vi "vision1.vi"(8 "error in":errorcluster) -> (0 "error out":errorcluster)   [LabVIEW 2017]
uses:
  <vilib>/userdefined/High Color/IMAQdx.ctl
  addres.vi
  <vilib>/vision/driver/NI_Vision_Acquisition_Software.lvlib
panel:
  out "color":string
  out "number":string
  out "Image":T1(plugin-control)
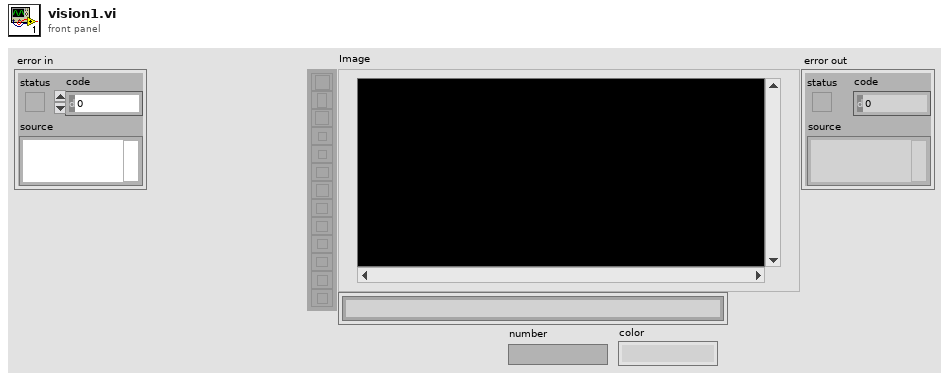
[diagram p1: front panel]
types:
  T1 = typedef "IMAQ Image.ctl" = refnum<image>
  T2 = typedef "IMAQdx.ctl" = refnum<k21>
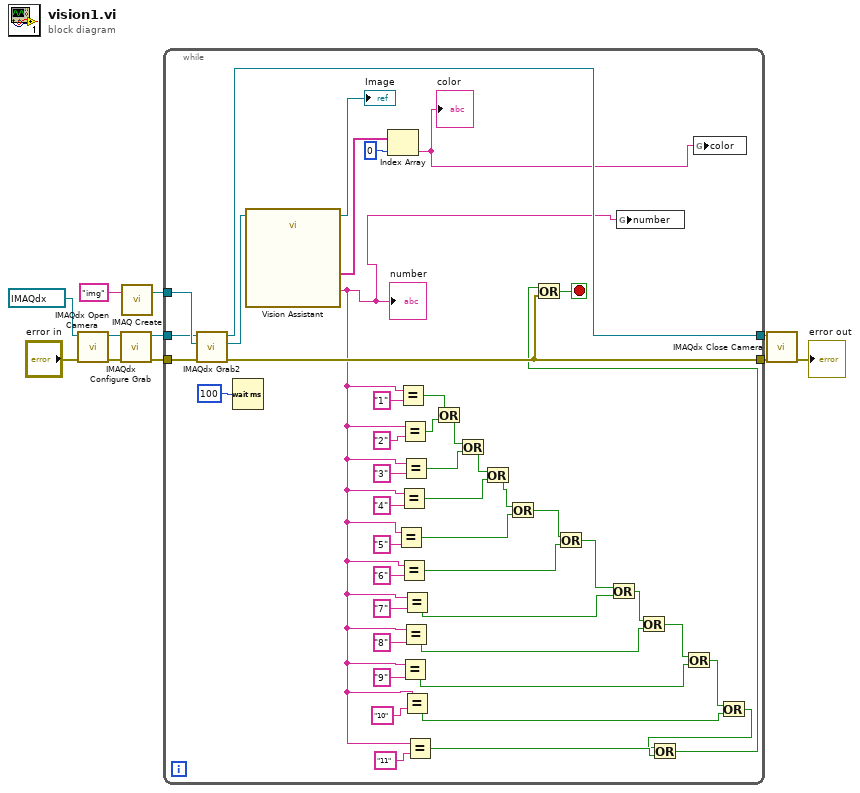
[diagram p0: block diagram]
diagram:
  n1 = call <vilib>:"IMAQdx Open Camera.vi"("error in"="error in", "Session In"=T2 "cam0") -> ("error out"=w8:errorcluster, "Session Out"=w5:T2)  [unwired: 8 in]
  n2 = call <vilib>:"IMAQdx Configure Grab.vi"("error in"=w8, "Session In"=w5) -> ("error out"=w7:errorcluster, "Session Out"=w4:T2)  [unwired: 8 in]
  n3 = call "IMAQ Create"("Image Name"="img") -> ("New Image"=w6:T1)  [unwired: 4 in, 1 out]
  n4 = while {
    tunnel: w7 -> [w56]
    tunnel: w6 -> [w55]
    tunnel: w4 -> [w54]
    tunnel: [w53] -> w3
    tunnel: [w47] -> w11
    stop <- w46 stop-if-true
    n5 = call <vilib>:"IMAQdx Grab2.vi"("error in"=w56, "Image In"=w55, "Session In"=w54) -> ("error out"=w47:errorcluster, "Image Out"=w52:T1, "Session Out"=w53:T2)  [unwired: 5 in, 1 out]
    n6 = Wait (ms)(milliseconds to wait=u32 100) -> ()  [unwired: 1 out]
    n7 = call "Vision Assistant"("Image In"=w52) -> ("Image Out"=→"Image":T1, "String (OCR/OCV 1)"=w15:string, "Classes (Color Classification 1)"=w49:string[])  [unwired: 23 in, 1 out]
    "number" <- w15
    n8 = Index Array(array=w49, index=0) -> (element=w17:string)
    "color" <- w17
    n9 = Equal?(x=w15, y="5") -> (x = y?=w35:bool)
    n10 = Equal?(x=w15, y="1") -> (x = y?=w28:bool)
    n11 = Equal?(x=w15, y="4") -> (x = y?=w33:bool)
    n12 = Equal?(x=w15, y="6") -> (x = y?=w37:bool)
    n13 = Equal?(x=w15, y="2") -> (x = y?=w29:bool)
    n14 = Equal?(x=w15, y="9") -> (x = y?=w43:bool)
    n15 = Equal?(x=w15, y="3") -> (x = y?=w31:bool)
    n16 = Equal?(x=w15, y="8") -> (x = y?=w40:bool)
    n17 = Equal?(x=w15, y="7") -> (x = y?=w39:bool)
    n18 = Equal?(x=w15, y="10") -> (x = y?=w45:bool)
    n19 = Equal?(x=w15, y="11") -> (x = y?=w14:bool)
    n20 = Or(x=w28, y=w29) -> (x .or. y?=w30:bool)
    n21 = Or(x=w30, y=w31) -> (x .or. y?=w32:bool)
    n22 = Or(x=w32, y=w33) -> (x .or. y?=w34:bool)
    n23 = Or(x=w34, y=w35) -> (x .or. y?=w36:bool)
    n24 = Or(x=w36, y=w37) -> (x .or. y?=w38:bool)
    n25 = Or(x=w38, y=w39) -> (x .or. y?=w41:bool)
    n26 = global write "addres.vi" "number"(w15) -> ()
    n27 = Or(x=w41, y=w40) -> (x .or. y?=w42:bool)
    n28 = Or(x=w42, y=w43) -> (x .or. y?=w44:bool)
    n29 = global write "addres.vi" "color"(w17) -> ()
    n30 = Or(x=w44, y=w45) -> (x .or. y?=w13:bool)
    n31 = Or(x=w13, y=w14) -> (x .or. y?=w12:bool)
    n32 = Or(x=w12, y=w47) -> (x .or. y?=w46:bool)
  }
  n33 = call <vilib>:"IMAQdx Close Camera.vi"("error in"=w11, "Session In"=w3) -> ("error out"=→"error out":errorcluster)  [unwired: 9 in]
